vi "Initialization (SubVI).vi"(0 "Trigger Level (% of Scale)":dbl=10.0 min=0.1 max=99.9 step=0.1 format="%_3f", 1 "VISA Refnum in":refnum<visa-resource-name>, 5 "Offset":sgl, 7 "Multiplier":sgl, 9 "Wavelength (nm)":u32=1064, 11 "error in":errorcluster, 12 "Scale":u32=999) -> (8 "VISA Refnum out":refnum<visa-resource-name>, 10 "error out":errorcluster)   [LabVIEW 2017]
doc: "by Tanguy BOULARD"
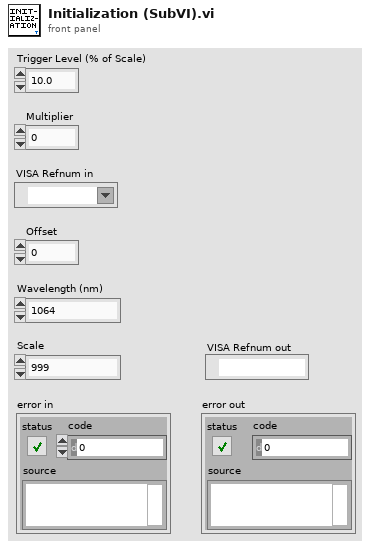
[diagram p1: front panel]
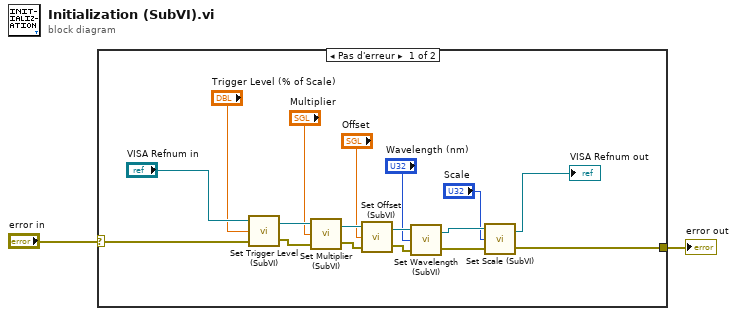
[diagram p0: block diagram]
diagram:
  n1 = case shown="Pas d'erreur" "error in" {
    selector: "error in" -> [w5 w20]
    tunnel: [w4 w20] -> w2
    frame No Error {
      n2 = call "Set Trigger Level (SubVI).vi"("error in"=w5, "Trigger Level (% of Scale)"="Trigger Level (% of Scale)", "VISA Refnum in"="VISA Refnum in") -> ("error out"=w13:errorcluster, "VISA Refnum out"=w17:refnum<visa-resource-name>)
      n3 = call "Set Multiplier (SubVI).vi"("error in"=w13, "Multiplier"="Multiplier", "VISA Refnum in"=w17) -> ("error out"=w14:errorcluster, "VISA Refnum out"=w18:refnum<visa-resource-name>)
      n4 = call "Set Offset (SubVI).vi"("error in"=w14, "Offset in"="Offset", "VISA Refnum in"=w18) -> ("error out"=w15:errorcluster, "VISA Refnum out"=w19:refnum<visa-resource-name>)
      n5 = call "Set Wavelength (SubVI).vi"("error in"=w15, "Wavelength (nm)"="Wavelength (nm)", "VISA Refnum in"=w19) -> ("error out"=w8:errorcluster, "VISA Refnum out"=w7:refnum<visa-resource-name>)
      n6 = call "Set Scale (SubVI).vi"("error in"=w8, "Scale"="Scale", "VISA Refnum in"=w7) -> ("error out"=w4:errorcluster, "VISA Refnum out"=→"VISA Refnum out":refnum<visa-resource-name>)
    }
    frame Error {
    }
  }
  "error out" <- w2
